vi "GT Get Lead Screw Comp Inner Value.vi"(6 "pCompValue":i32, 7 "pos":i32, 8 "error in (no error)":errorcluster caption="错误输入（无错误）", 9 "dir":i16, 10 "axis":i16, 11 "cardNum":i16) -> (0 "error out":errorcluster caption="错误输出", 3 "function return":i16, 4 "pCompValue out":i32)   [LabVIEW 2014, in "gts.lvlib"]
doc: "GT_API GT_GetLeadScrewCompInnerValue(short cardNum,short axis,short dir,long pos,long *pCompValue);"
uses:
  gts.lvlib
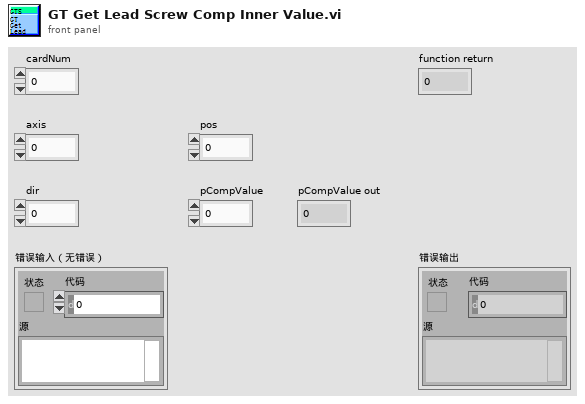
[diagram p1: front panel]
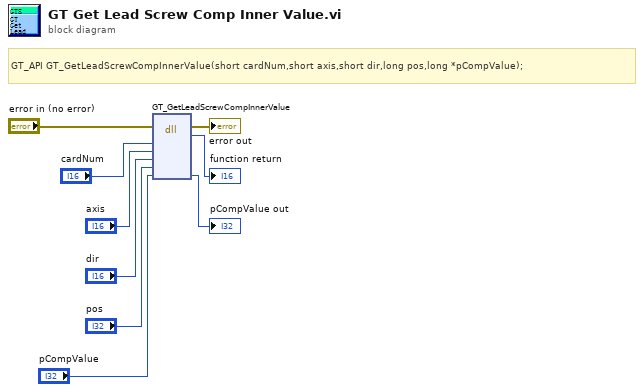
[diagram p0: block diagram]
diagram:
  # "GT_API GT_GetLeadScrewCompInnerValue(short cardNum,short axis,short dir,long pos,long *pCompValue);"
  n1 = dll-call lib="PTH2habs D固高科技资料GTS控制卡GTS卡18年上半年资料dllVC32bit\nmulti_cardgts.*" fn="GT_GetLeadScrewCompInnerValue"(error in="error in (no error)", "cardNum"="cardNum", "axis"="axis", "dir"="dir", "pos"="pos", "pCompValue"="pCompValue") -> (error out=→"error out":errorcluster, →"function return":i16, "pCompValue"=→"pCompValue out":i32)  [unwired: 6 in, 1 out]
